vi "subFrameSyncandFreqOffset.vi"(0 "Data stream":cdb[][](array[numeric]), 9 "System Parameters":T1={"Symbol Rate"=64.0, "Symbols per Packet"=8, "Tx Oversample Factor"=16, "Rx Oversample Factor"=16, "Modulation Scheme"=enum."4-QAM", "filter length (symbols)"=8, "filter parameter"=0.5, "Training Sequence"=[], "Channel Length Estimate"=4, "Frequency Offset\nCorrection?"=TRUE} {"Symbol Rate" format="%#_6p"; "Training Sequence" format="%#_3p"; "filter parameter" format="%.2f"}, 11 "error in (no error)":errorcluster) -> (4 "Data stream (out)":cdb[][](array[numeric]), 6 "frequency offsets":dbl[](array[numeric]), 8 "frame offset":i32, 10 "System Parameters (out)":T1={"Symbol Rate"=64.0, "Symbols per Packet"=8, "Tx Oversample Factor"=16, "Rx Oversample Factor"=16, "Modulation Scheme"=enum."4-QAM", "filter length (symbols)"=8, "filter parameter"=0.5, "Training Sequence"=[], "Channel Length Estimate"=4, "Frequency Offset\nCorrection?"=TRUE} {"Symbol Rate" format="%#_6p"; "Training Sequence" format="%#_3p"; "filter parameter" format="%.2f"}, 15 "error out":errorcluster)   [LabVIEW 2011]
uses:
  ModulationParameters.ctl
panel:
  out "antenna index used for sync":i32
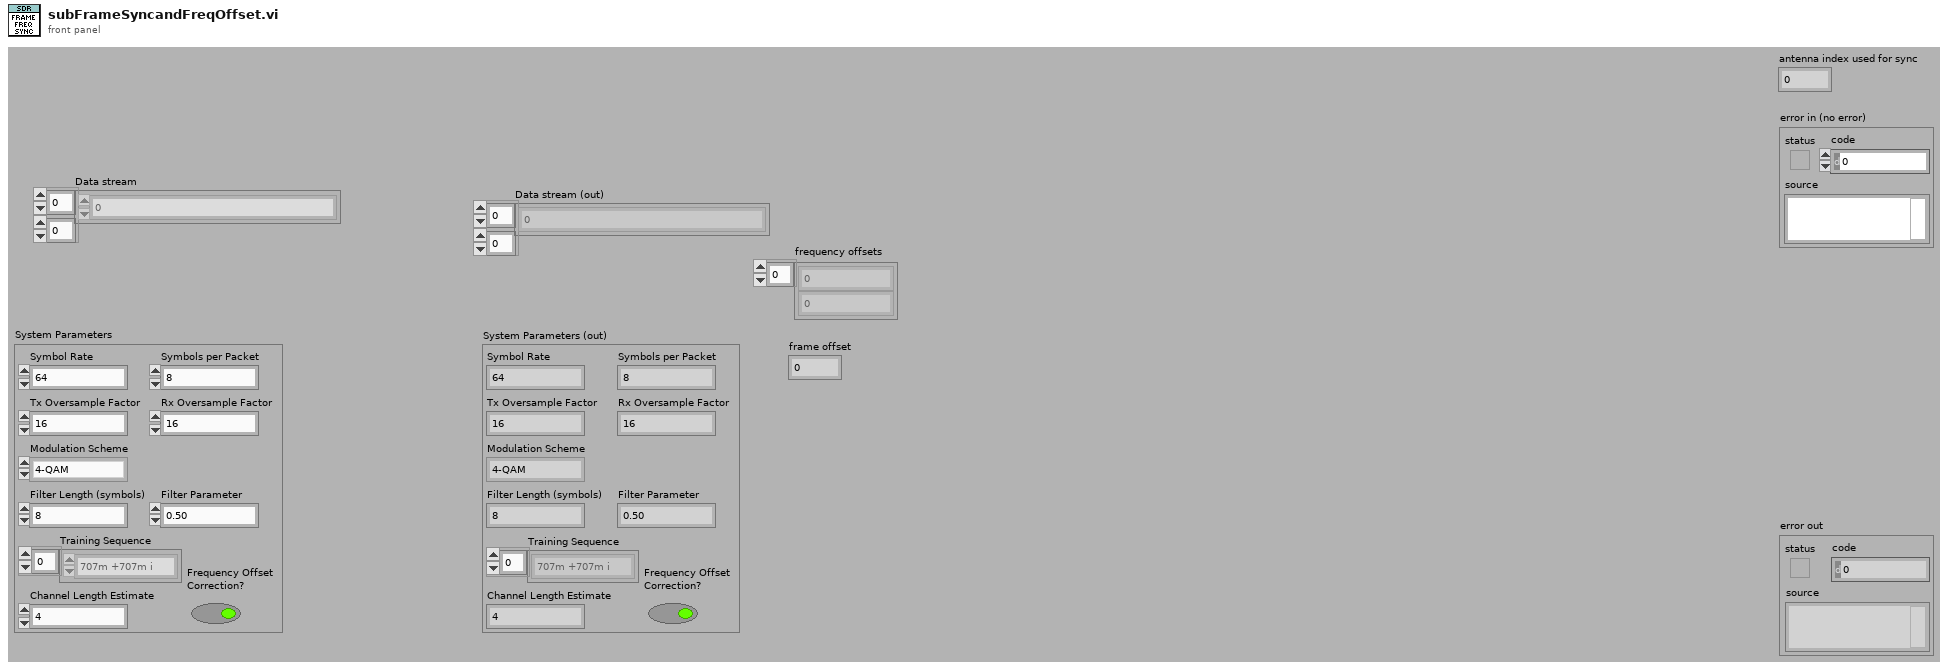
[diagram p1: front panel]
types:
  T1 = typedef "ModulationParameters.ctl" = cluster{"Symbol Rate":dbl, "Symbols per Packet":i32, "Tx Oversample Factor":i32, "Rx Oversample Factor":i32, "Modulation Scheme":enum16{"4-QAM", "16-QAM", "64-QAM"}, "filter length (symbols)":i32, "filter parameter":dbl, "Training Sequence":cdb[], "Channel Length Estimate":i32, "Frequency Offset\nCorrection?":bool}
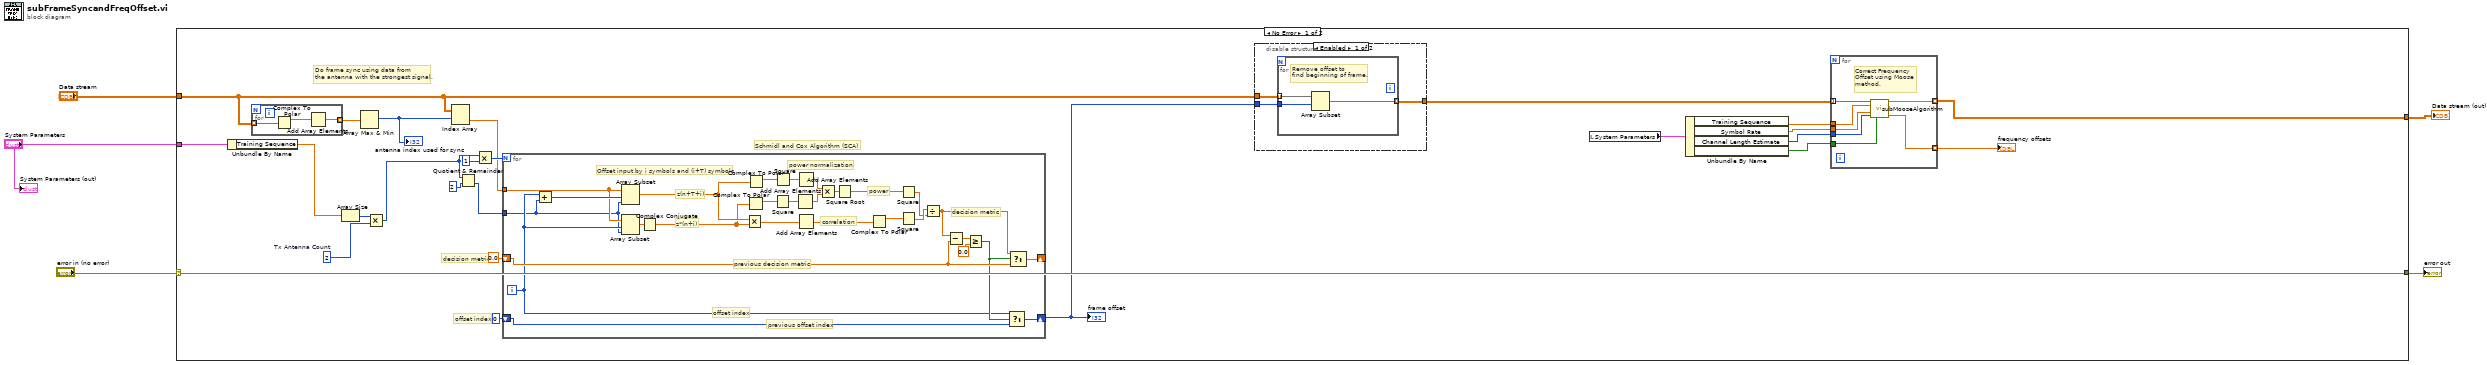
[diagram p0: block diagram]
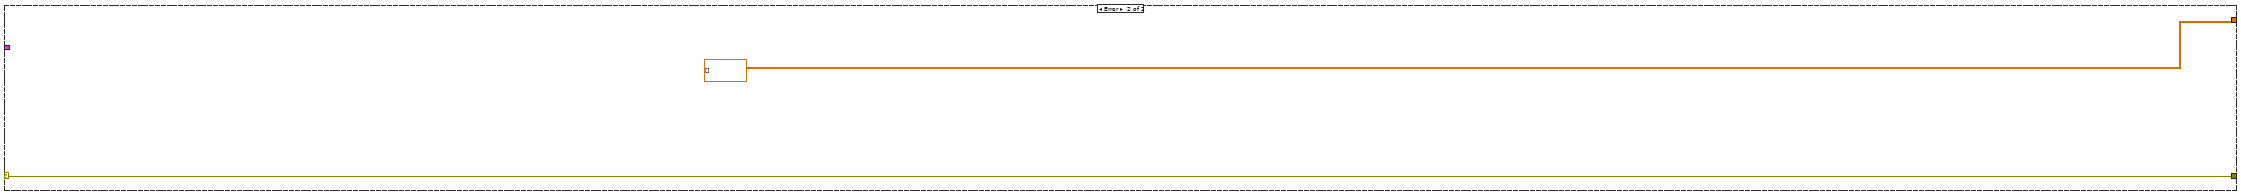
[diagram p3: hidden frame]
diagram:
  n1 = case shown="No Error" "error in (no error)" {
    selector: "error in (no error)" -> [w22 w77]
    tunnel: [w22 w77] -> w4
    tunnel: "Data stream" -> [w8 _]
    tunnel: "System Parameters" -> [w30 _]
    tunnel: [w7 cdb[][] [] ("output")] -> w1
    frame No Error {
      w6 = 2  # Tx Antenna Count
      # "Schmidl and Cox Algorithm (SCA)"
      # "decision metric"
      # "offset index"
      # "Do frame sync using data from \nthe antenna with the strongest signal."
      n2 = Unbundle By Name(w30) -> ("Training Sequence"=w12:cdb[])
      n3 = for {
        tunnel: w8 -> [w68] mode=indexing
        tunnel: [w66] -> w21 mode=indexing
        n4 = Complex To Polar(r * e^(i*theta)=w68) -> (r=w67:dbl[])  [unwired: 1 out]
        n5 = Add Array Elements(numeric array=w67) -> (sum=w66:dbl)
      }
      n6 = Array Size(array=w12) -> (size(s)=w11:i32)
      n7 = Array Max & Min(array=w21) -> (max index (indices)=w13:i32)  [unwired: 3 out]
      "antenna index used for sync" <- w13
      n8 = Multiply(x=w11, y=w6) -> (x*y=w10:i32)
      n9 = Index Array(array=w8, index (row)=w13) -> (element=w14:cdb[])  [unwired: 1 in]
      n10 = Quotient & Remainder(x=w10, y=2) -> (floor(x/y)=w17:i32)  [unwired: 1 out]
      n11 = Multiply(x=w10, y=1) -> (x*y=w19:i32)
      n12 = for {
        N: w19 -> [_]
        tunnel: w17 -> [w47]
        shift-right: [w64] -> _
        shift-left: 0.0 -> [w60]
        shift-right: [w65] -> w9
        shift-left: 0 -> [w59]
        tunnel: w14 -> [w49]
        i -> [w48]
        # "power"
        # "offset index"
        # "previous offset index"
        # "previous decision metric"
        # "decision metric"
        # "power normalization"
        # "correlation"
        # "Offset input by i symbols and (i+T) symbols"
        # "z(n+T+i)"
        # "z*(n+i)"
        n13 = Add(x=w48, y=w47) -> (x+y=w57:i32)
        n14 = Array Subset(array=w49, index=w57, length=w47) -> (w61:cdb[])
        n15 = Array Subset(array=w49, index=w48, length=w47) -> (w62:cdb[])
        n16 = Complex Conjugate(1:w62) -> (0:w42:cdb[])
        n17 = Multiply(x=w61, y=w42) -> (x*y=w56:cdb[])
        n18 = Complex To Polar(r * e^(i*theta)=w42) -> (r=w44:dbl[])  [unwired: 1 out]
        n19 = Complex To Polar(r * e^(i*theta)=w61) -> (r=w54:dbl[])  [unwired: 1 out]
        n20 = Square(x=w44) -> (x^2=w43:dbl[])
        n21 = Square(x=w54) -> (x^2=w55:dbl[])
        n22 = Add Array Elements(numeric array=w43) -> (sum=w41:dbl)
        n23 = Add Array Elements(numeric array=w55) -> (sum=w39:dbl)
        n24 = Add Array Elements(numeric array=w56) -> (sum=w58:cdb)
        n25 = Multiply(x=w39, y=w41) -> (x*y=w40:dbl)
        n26 = Square Root(x=w40) -> (sqrt(x)=w38:dbl)
        n27 = Complex To Polar(r * e^(i*theta)=w58) -> (r=w50:dbl)  [unwired: 1 out]
        n28 = Square(x=w38) -> (x^2=w45:dbl)
        n29 = Square(x=w50) -> (x^2=w46:dbl)
        n30 = Divide(x=w46, y=w45) -> (x/y=w63:dbl)
        n31 = Subtract(x=w63, y=w60) -> (x-y=w51:dbl)
        n32 = Greater Or Equal?(x=w51, y=0.0 ("1/x")) -> (x >= y?=w52:bool)
        n33 = Select(t=w48, s=w52, f=w59) -> (s? t:f=w65:i32)
        n34 = Select(t=w63, s=w52, f=w60) -> (s? t:f=w64:dbl)
      }
      "frame offset" <- w9
      n35 = disable-structure shown="Enabled" {
        disable-tunnel: [w33 w37] -> w28
        disable-tunnel: w9 -> [w32 _]
        disable-tunnel: w8 -> [w31 w37]
        frame Enabled {
          n36 = for {
            tunnel: [w34] -> w33 mode=indexing
            tunnel: w32 -> [w36]
            tunnel: w31 -> [w35] mode=indexing
            # "Remove offset to \nfind beginning of frame."
            n37 = Array Subset(array=w35, index=w36) -> (w34:cdb[])  [unwired: 1 in]
          }
        }
        frame Disabled {
        }
      }
      n38 = local read "System Parameters"() -> (w29:T1)
      n39 = Unbundle By Name(w29) -> ("Training Sequence"=w27:cdb[], "Symbol Rate"=w23:dbl, "Channel Length Estimate"=w26:i32, "Frequency Offset\nCorrection?"=w25:bool)
      n40 = for {
        tunnel: w28 -> [w69] mode=indexing
        tunnel: w27 -> [w75]
        tunnel: w23 -> [w74]
        tunnel: w26 -> [w73]
        tunnel: [w72] -> w7 mode=indexing
        tunnel: w25 -> [w71]
        tunnel: [w70] -> w24 mode=indexing
        # "Correct Frequency \nOffset using Moose\nmethod."
        n41 = call "subMooseAlgorithm.vi"("input"=w69, "Training Sequence"=w75, "symbol rate"=w74, "channel estimate length"=w73, "Correct Frequency Offset?"=w71) -> ("output"=w72:cdb[], "frequency offset (Hz)"=w70:dbl)  [unwired: 9 in]
      }
      "frequency offsets" <- w24
    }
    frame Error {
    }
  }
  "error out" <- w4
  "Data stream (out)" <- w1
  "System Parameters (out)" <- "System Parameters"
